vi "test Get PCAN API Version.vi"(11 "Test Case In":refnum<class "Test PCANBasic.lvclass">) -> (0 "error out":errorcluster, 3 "Test Case Out":refnum<class "Test PCANBasic.lvclass">)   [LabVIEW 2020, in "Test PCANBasic.lvclass"]
uses:
  Test PCANBasic.lvclass
  Test PCANBasic.lvclass/Test PCANBasic.ctl
  <vilib>/Astemes/LUnit/Test Case.lvclass
  source/PCANBasic.lvlib
  source/Get PCAN API Version.vi
panel:
  out "Channel Version":string
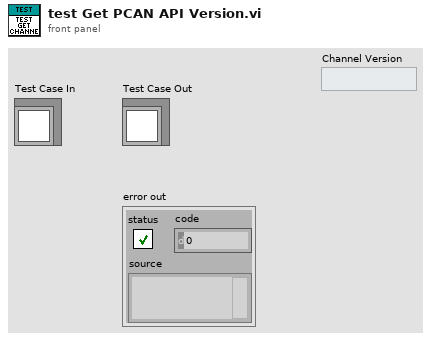
[diagram p1: front panel]
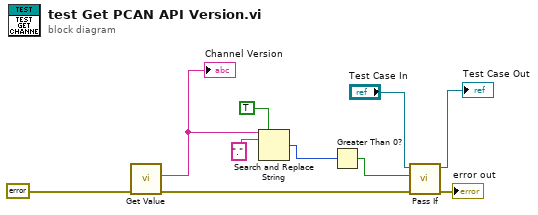
[diagram p0: block diagram]
diagram:
  n1 = call-poly "Get Value.vi"("error in"=errorcluster {"status"=FALSE, "code"=0, "source"=""}) -> ("error out"=w6:errorcluster, "PCAN API Version"=w3:string)  [unwired: 8 in, 1 out]
  "Channel Version" <- w3
  n2 = Search and Replace String(replace all?=TRUE ("replace all? (F)"), input string=w3, search string=".") -> (number of replacements=w1:i32)  [unwired: 5 in, 3 out]
  n3 = Greater Than 0?(x=w1) -> (x > 0?=w2:bool)
  n4 = call <vilib>:"Pass If.vi"("error in (no error)"=w6, "Pass?"=w2, "LUnit Test Case In"="Test Case In") -> ("error out"=→"error out":errorcluster, "LUnit Test Case Out"=→"Test Case Out":refnum<class "Test PCANBasic.lvclass">)  [unwired: 7 in]
